vi "Parse String to Array_Int.vi"(6 "Spliter 2":string, 11 "String Input":string) -> (2 "Data 2":i32[][](array[numeric]), 3 "Data 1":i32[](array[numeric]))   [LabVIEW 2020, in "GUCalibration2.lvlib"]
uses:
  GUCalibration2.lvlib
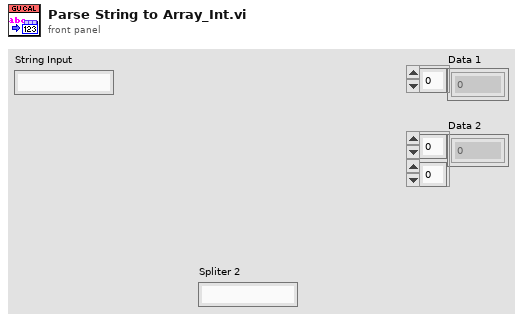
[diagram p1: front panel]
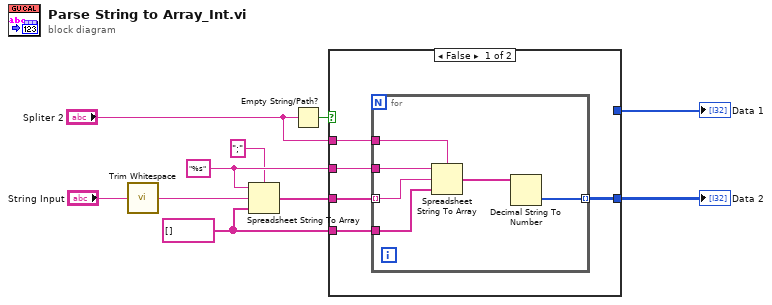
[diagram p0: block diagram]
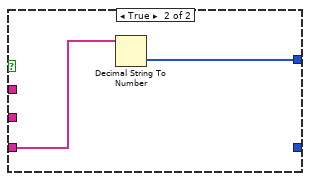
[diagram p2: hidden frame]
diagram:
  w2 = "%s" ("format string")
  w4 = string[] []
  n1 = call <vilib>:"Trim Whitespace.vi"("string"="String Input") -> ("trimmed string"=w3:string)  [unwired: 1 in]
  n2 = Spreadsheet String To Array(delimiter (Tab)=";" ("format string"), format string=w2, spreadsheet string=w3, array type (2D Dbl)=w4) -> (array=w5:string[])
  n3 = Empty String/Path?(string/path="Spliter 2") -> (empty?=w6:bool)
  n4 = case shown="False" w6 {
    tunnel: w5 -> [w15 w23]
    tunnel: "Spliter 2" -> [w14 _]
    tunnel: w4 -> [w13 _]
    tunnel: w2 -> [w12 _]
    tunnel: [w11 _] -> w8
    tunnel: [_ w22] -> w7
    frame False {
      n5 = for {
        tunnel: w15 -> [w19] mode=indexing
        tunnel: w14 -> [w20]
        tunnel: w13 -> [w21]
        tunnel: w12 -> [w18]
        tunnel: [w16] -> w11 mode=indexing
        n6 = Spreadsheet String To Array(delimiter (Tab)=w20, format string=w18, spreadsheet string=w19, array type (2D Dbl)=w21) -> (array=w17:string[])
        n7 = Decimal String To Number(string=w17) -> (number=w16:i32[])  [unwired: 2 in, 1 out]
      }
    }
    frame True {
      n8 = Decimal String To Number(string=w23) -> (number=w22:i32[])  [unwired: 2 in, 1 out]
    }
  }
  "Data 2" <- w8
  "Data 1" <- w7
